vi "Value DBL.vi"(8 "error in (no error)":errorcluster, 10 "Hierarchy":string[](array[string]), 11 "Config Manager in":refnum<class "Config Manager.lvclass">) -> (0 "error out":errorcluster, 2 "DBL Value":dbl, 3 "Config Manager out":refnum<class "Config Manager.lvclass">)   [LabVIEW 2020, in "CDM-Config.lvlib" / "Config Manager.lvclass"]
uses:
  Config Manager.lvclass
  Config Element/Config Element.lvclass
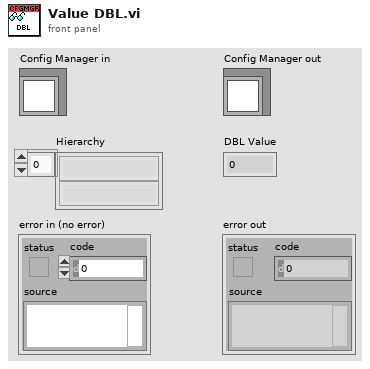
[diagram p1: front panel]
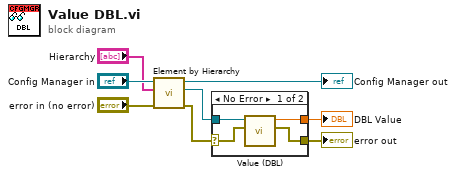
[diagram p0: block diagram]
diagram:
  n1 = call "Element by Hierarchy.vi"("error in (no error)"="error in (no error)", "Hierarchy"="Hierarchy", "Config Manager in"="Config Manager in") -> ("error out"=w2:errorcluster, "Config Element"=w1:refnum<class "Config Element.lvclass">, "Config Manager out"=→"Config Manager out":refnum<class "Config Manager.lvclass">)  [unwired: 6 in]
  n2 = case shown="No Error" w2 {
    selector: w2 -> [w10 w13]
    tunnel: w1 -> [w12 _]
    tunnel: [w9 w13] -> w8
    tunnel: [w11 _] -> w7
    frame No Error {
      n3 = call "Value (DBL).vi"("error in (no error)"=w10, "Config Element in"=w12) -> ("error out"=w9:errorcluster, "DBL Value"=w11:dbl)  [unwired: 8 in]
    }
    frame Error {
    }
  }
  "error out" <- w8
  "DBL Value" <- w7
